vi "T12 - Одиночное измерение.vi"() -> ()   [LabVIEW 2009]
uses:
  Z210/Z210 CTL Lib.llb/Z210 CTL ADC Voltages.ctl
  Z210/Z210 CTL Lib.llb/Z210 CTL DAC Voltages.ctl
  Z210/Z210 CTL Lib.llb/Z210 CTL ADC Linear Correction.ctl
  Z210/Z210 CTL Lib.llb/Z210 CTL ADC or DAC Function.ctl
panel:
  in  "Linear Correction ADC":T1=[{"scale"=1.0, "offset"=0.0}, {"scale"=1.0, "offset"=0.0}, {"scale"=1.0, "offset"=0.0}, {"scale"=1.0, "offset"=0.0}, {"scale"=1.0, "offset"=0.0}, {"scale"=1.0, "offset"=0.0}, {"scale"=1.0, "offset"=0.0}, {"scale"=1.0, "offset"=0.0}, {"scale"=1.0, "offset"=0.0}, {"scale"=1.0, "offset"=0.0}, {"scale"=1.0, "offset"=0.0}, {"scale"=1.0, "offset"=0.0}, {"scale"=1.0, "offset"=0.0}, {"scale"=1.0, "offset"=0.0}, {"scale"=1.0, "offset"=0.0}, {"scale"=1.0, "offset"=0.0}]
  in  "DAC Voltages":T2=[1.0, 2.0]
  in  "delay (100)":i32=100
  out "ADC Voltages":T3
  # "1. Соединить:\n    • DAC#0 <-> ADC#0\n    • DAC#1 <-> ADC#1\n2. Задать коэффициенты коорекции по вкусу.\n3. ...\n4. PROFIT"
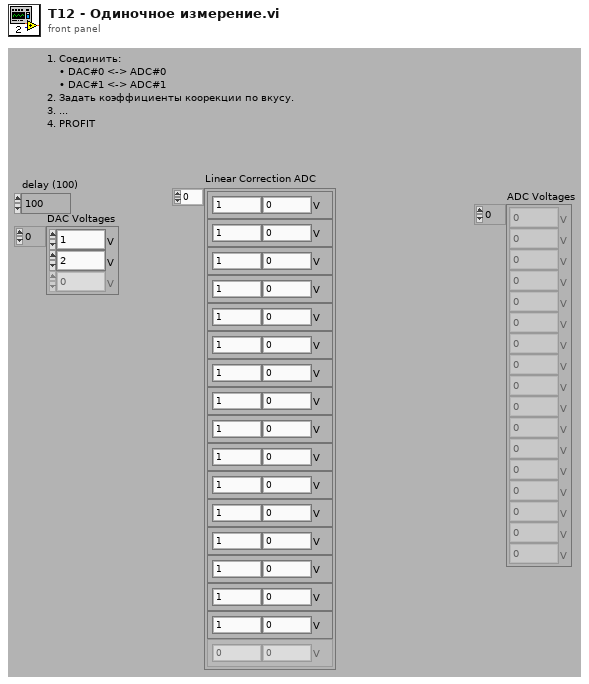
[diagram p1: front panel]
types:
  T1 = typedef "Z210 CTL ADC Linear Correction.ctl" = cluster{"scale":dbl, "offset":dbl[unit]}[]
  T2 = typedef "Z210 CTL DAC Voltages.ctl" = dbl[unit][]
  T3 = typedef "Z210 CTL ADC Voltages.ctl" = dbl[unit][]
  T4 = typedef "Z210 CTL ADC or DAC Function.ctl" = enum16{"АЦП", "ЦАП", "Both"}
  T5 = typedef "Z210 CTL Unit Data .ctl" = cluster{"typeDevice":i32, "numberDSP":i32}
  T6 = typedef "Z210 CTL Buffers Params.ctl" = cluster{"bufferAddr ADC":u32, "bufferSize ADC":i32, "bufferAddr DAC":u32, "bufferSize DAC":i32}
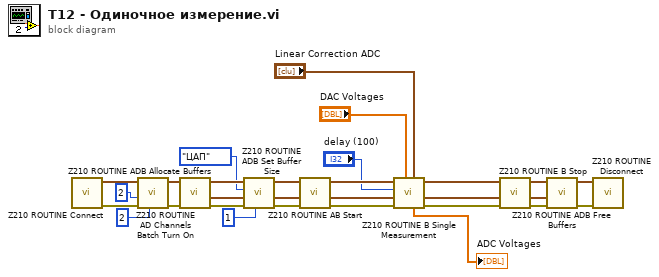
[diagram p0: block diagram]
diagram:
  n1 = call "Z210 ROUTINE Connect.vi"() -> ("error out"=w28:errorcluster, "unitData out"=w29:T5)  [unwired: 10 in]
  n2 = call "Z210 ROUTINE AD Channels Batch Turn On.vi"("N ЦАП (0)"=2, "error in (no error)"=w28, "N Синф (0)"=2, "unitData in"=w29) -> ("error out"=w26:errorcluster, "unitData out"=w27:T5)  [unwired: 4 in, 2 out]
  n3 = call "Z210 ROUTINE ADB Allocate Buffers.vi"("error in (no error)"=w26, "unitData in"=w27) -> ("error out"=w20:errorcluster, "buffersParams out"=w23:T6, "unitData out"=w22:T5)  [unwired: 7 in]
  n4 = call "Z210 ROUTINE ADB Set Buffer Size.vi"("size suggestion (0)"=1, "error in (no error)"=w20, "buffersParams"=w23, "AorD"=Z210_CTL_ADC_or_DAC_Function."ЦАП", "unitData in"=w22) -> ("error out"=w17:errorcluster, "buffersParams out"=w16:T6, "unitData out"=w18:T5)  [unwired: 4 in]
  n5 = call "Z210 ROUTINE AB Start.vi"("error in (no error)"=w17, "buffersParams"=w16, "unitData in"=w18) -> ("error out"=w9:errorcluster, "buffersParams out"=w8:T6, "unitData out"=w10:T5)  [unwired: 6 in]
  n6 = call "Z210 ROUTINE B Single Measurement.vi"("Linear Correction ADC"="Linear Correction ADC", "DAC Voltages"="DAC Voltages", "error in (no error)"=w9, "buffersParams"=w8, "delay (100)"="delay (100)", "unitData in"=w10) -> ("error out"=w2:errorcluster, "buffersParams out"=w3:T6, "unitData out"=w4:T5, "ADC Voltages"=→"ADC Voltages":T3)  [unwired: 2 in]
  n7 = call "Z210 ROUTINE B Stop.vi"("error in (no error)"=w2, "buffersParams"=w3, "unitData in"=w4) -> ("error out"=w13:errorcluster, "buffersParams out"=w14:T6, "unitData out"=w15:T5)  [unwired: 6 in]
  n8 = call "Z210 ROUTINE ADB Free Buffers.vi"("error in (no error)"=w13, "buffersParams"=w14, "unitData in"=w15) -> ("error out"=w11:errorcluster, "unitData out"=w12:T5)  [unwired: 6 in, 1 out]
  n9 = call "Z210 ROUTINE Disconnect.vi"("error in (no error)"=w11, "unitData in"=w12) -> ()  [unwired: 8 in, 2 out]
